vi "accelerometer_real_data.vi"(2 "speed subarray":dbl[](array[numeric]), 3 "transposed array":dbl[][](array[numeric]), 4 "x,y,z?":i32=1, 5 "Speed Index":i32) -> (0 "Speed":dbl, 1 "Accleration Array":dbl[](array[numeric]))   [LabVIEW 2025]
uses:
  468687ae-6b61-4150-b139-1e5540973179.vi
panel:
  # "Data from: https://data.mendeley.com/datasets/5rrxw7y5bj/1"
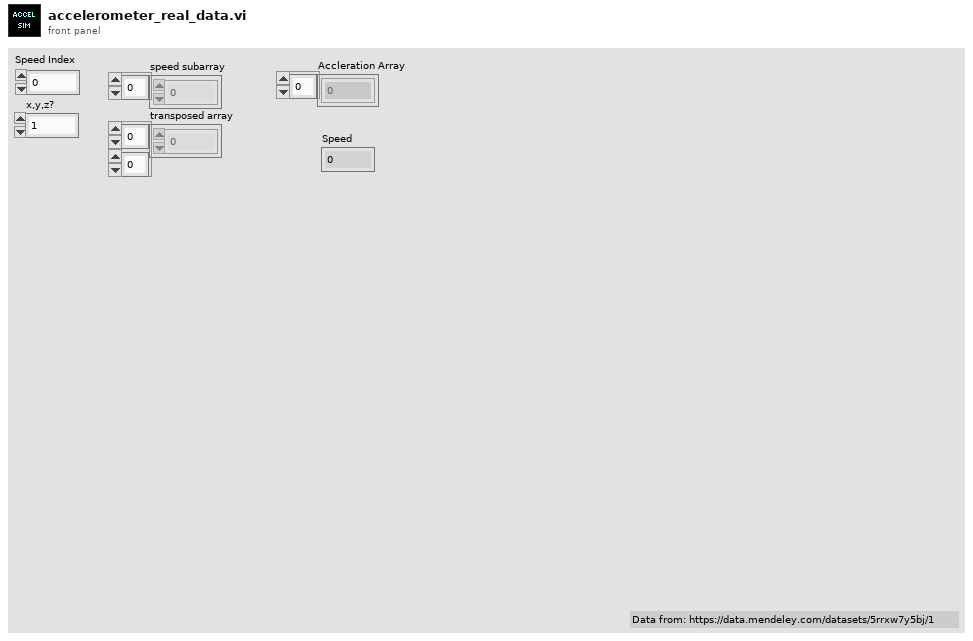
[diagram p1: front panel]
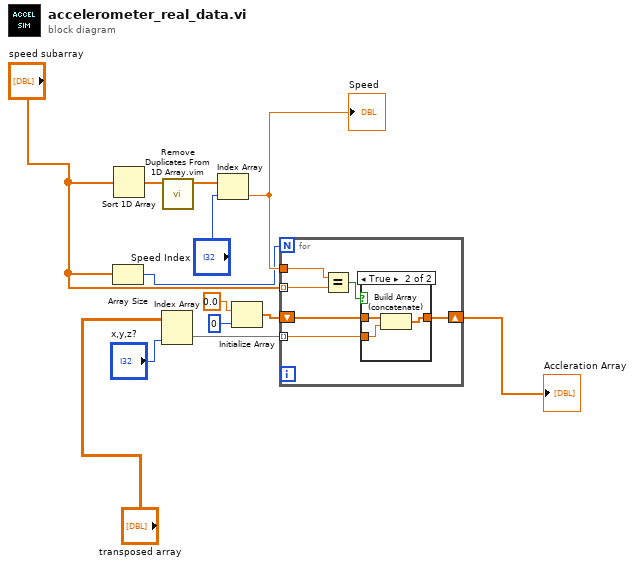
[diagram p0: block diagram]
diagram:
  n1 = Array Size(array="speed subarray") -> (size(s)=w9:i32)
  n2 = Sort 1D Array(array="speed subarray") -> (sorted array=w6:dbl[])
  n3 = Index Array(array="transposed array", index (col)="x,y,z?") -> (element=w13:dbl[])  [unwired: 1 in]
  n4 = call "Remove Duplicates From 1D Array.vim"("array"=w6) -> ("array with duplicates removed"=w8:dbl[])  [unwired: 10 in]
  n5 = Index Array(array=w8, index="Speed Index") -> (element=w10:dbl)
  "Speed" <- w10
  n6 = Initialize Array(0.0 ("element"), 0 ("dimension size")) -> (w11:dbl[])
  n7 = for {
    N: w9 -> [_]
    tunnel: "speed subarray" -> [w16] mode=indexing
    tunnel: w10 -> [w19]
    shift-right: [w14] -> w3
    shift-left: w11 -> [w17]
    tunnel: w13 -> [w15] mode=indexing
    n8 = Equal?(x=w19, y=w16) -> (x = y?=w18:bool)
    n9 = case shown="True" w18 {
      tunnel: w17 -> [w20 w23]
      tunnel: [w20 w22] -> w14
      tunnel: w15 -> [_ w21]
      frame False {
      }
      frame True {
        n10 = Build Array (concatenate)(w23, w21) -> (w22:dbl[])
      }
    }
  }
  "Accleration Array" <- w3
